vi "Get Instruments.vi"(8 "error in":errorcluster, 10 "Engine":string, 11 "Submodule in":refnum<class "Submodule EOL.lvclass">) -> (0 "error out":errorcluster, 1 "Instrument nodes":refnum<data-value>[](array[refnum]), 2 "Instruments":string[](array[string]), 3 "Submodule out":refnum<class "Submodule EOL.lvclass">)   [LabVIEW 2025, in "Submodule EOL.lvlib" / "Submodule EOL.lvclass"]
uses:
  Submodule EOL.lvclass
  Users/Public/Documents/Sandia National Labs/TSS Plugin/Abstract Engine.lvlibp/Plugin/Abstract/Abstract Instrument/Abstract Instrument.lvclass
  Users/Public/Documents/Sandia National Labs/TSS Plugin/Abstract Engine.lvlibp/Plugin/Abstract/Abstract Engine/Abstract Engine.lvclass
  Users/Public/Documents/Sandia National Labs/TSS Plugin/Abstract Engine.lvlibp/Plugin/Abstract/Engine configuration/Engine configuration.lvclass
  Users/Public/Documents/Sandia National Labs/TSS Plugin/Abstract Engine.lvlibp/Plugin/Abstract/Instrument configuration/Instrument configuration.lvclass
  Users/Public/Documents/Sandia National Labs/TSS Plugin/CEF.lvlibp/Node/ReadParent.vi
  Users/Public/Documents/Sandia National Labs/TSS Plugin/CEF.lvlibp/Node/ReadChildren.vi
  Users/Public/Documents/Sandia National Labs/TSS Plugin/CEF.lvlibp/Node/ReadNodeClass.vi
  Users/Public/Documents/Sandia National Labs/TSS Plugin/Abstract Engine.lvlibp/Plugin/Abstract/Engine configuration/Read Engine Setting.vi
  Users/Public/Documents/Sandia National Labs/TSS Plugin/Abstract Engine.lvlibp/Plugin/Abstract/Instrument configuration/Read Instrument Setting.vi
  Users/Public/Documents/Sandia National Labs/TSS Plugin/CEF.lvlibp/Node/CEF_Node.lvclass
  Users/Public/Documents/Sandia National Labs/TSS Plugin/CEF.lvlibp/serializable configuration/CEF_serializable configuration.lvclass
  Submodule EOL.lvclass/Submodule EOL.ctl
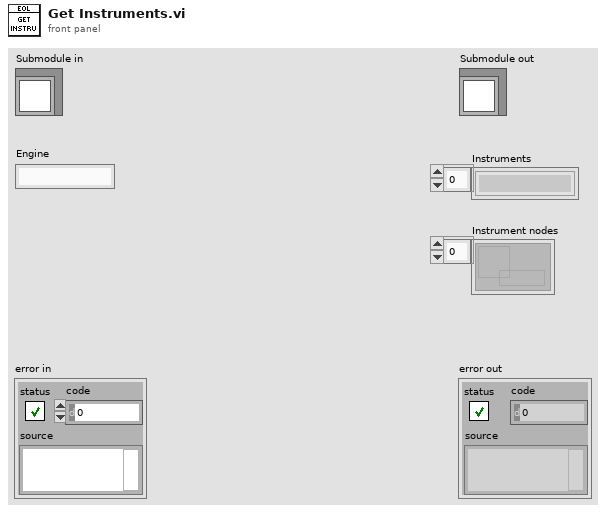
[diagram p1: front panel]
types:
  T1 = typedef "Abstract Engine.lvlibp/Engine configuration.lvclass/Engine Setting.ctl" = cluster{"Enabled":bool, "IP Address":string, "Port":i32, "Description":string, "Type":string, "Version":string}
  T2 = typedef "Abstract Engine.lvlibp/Instrument configuration.lvclass/Default Instrument.ctl" = cluster{"Type":string, "Address":string, "SW Alias":string, "Description":string, "Enabled":bool}
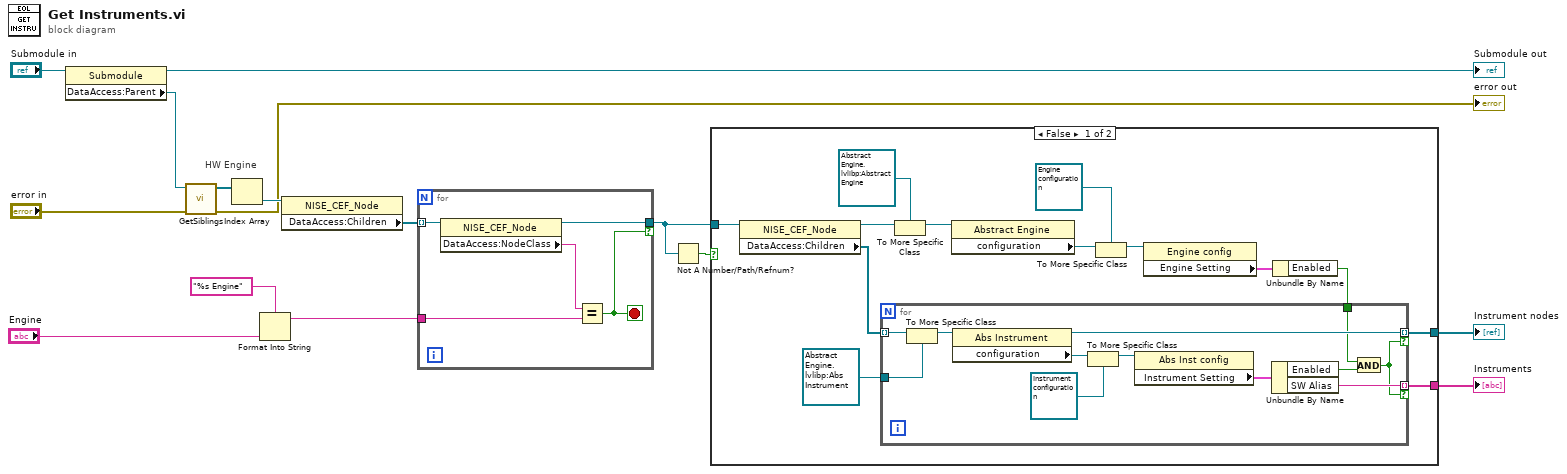
[diagram p0: block diagram]
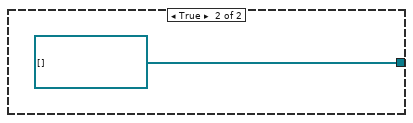
[diagram p2: hidden frame]
diagram:
  # "HW Engine"
  n1 = property class="Submodule"(reference="Submodule in") -> (reference out=→"Submodule out":refnum<class "Submodule EOL.lvclass">, "DataAccess:Parent"=w13:refnum<data-value>)  [unwired: 1 in, 1 out]
  n2 = call "GetSiblings.vi"("error in"="error in", "node in"=w13) -> ("error out"=→"error out":errorcluster, "siblings"=w12:refnum<data-value>[])  [unwired: 8 in]
  n3 = Index Array(array=w12) -> (element=w11:refnum<data-value>)  [unwired: 1 in]
  n4 = Format Into String(format string="%s Engine", "Engine") -> (resulting string=w1:string)  [unwired: 2 in, 1 out]
  n5 = property class="NISE_CEF_Node"(reference=w11) -> ("DataAccess:Children"=w10:refnum<data-value>[])  [unwired: 1 in, 2 out]
  n6 = for {
    tunnel: w10 -> [w20] mode=indexing
    tunnel: [w18] -> w8 if=w17
    tunnel: w1 -> [w16]
    stop <- w17 stop-if-true
    n7 = property class="NISE_CEF_Node"(reference=w20) -> (reference out=w18:refnum<data-value>, "DataAccess:NodeClass"=w19:string)  [unwired: 1 in, 1 out]
    n8 = Equal?(x=w19, y=w16) -> (x = y?=w17:bool)
  }
  n9 = Not A Number/Path/Refnum?(number/path/refnum=w8) -> (NaN/Path/Refnum?=w9:bool)
  n10 = case shown="False" w9 {
    tunnel: w8 -> [w33 _]
    tunnel: [w22 refnum<data-value>[] []] -> w6
    tunnel: [w21 _] -> w4
    frame False {
      n11 = property class="NISE_CEF_Node"(reference=w33) -> (reference out=w32:refnum<data-value>, "DataAccess:Children"=w30:refnum<data-value>[])  [unwired: 1 in, 1 out]
      n12 = To More Specific Class(target class=refnum<data-value> refnum, reference=w32) -> (specific class reference=w24:refnum<data-value>)  [unwired: 1 in, 1 out]
      n13 = property class="Abstract Engine"(reference=w24) -> ("configuration"=w28:refnum<class "CEF_serializable configuration.lvclass">)  [unwired: 1 in, 2 out]
      n14 = To More Specific Class(target class=refnum<class "Engine configuration.lvclass"> refnum ("Abstract Engine.lvlibp:Engine config"), reference=w28) -> (specific class reference=w27:refnum<class "Engine configuration.lvclass">)  [unwired: 1 in, 1 out]
      n15 = property class="Engine config"(reference=w27) -> ("Engine Setting"=w26:T1)  [unwired: 1 in, 2 out]
      n16 = Unbundle By Name(w26) -> ("Enabled"=w23:bool)
      n17 = for {
        tunnel: w30 -> [w45] mode=indexing
        tunnel: refnum<data-value> refnum ("target class") -> [w44]
        tunnel: [w38] -> w21 mode=indexing if=w34
        tunnel: [w37] -> w22 mode=indexing if=w34
        tunnel: w23 -> [w36]
        n18 = To More Specific Class(target class=w44, reference=w45) -> (specific class reference=w43:refnum<data-value>)  [unwired: 1 in, 1 out]
        n19 = property class="Abs Instrument"(reference=w43) -> (reference out=w37:refnum<data-value>, "configuration"=w42:refnum<class "CEF_serializable configuration.lvclass">)  [unwired: 1 in, 1 out]
        n20 = To More Specific Class(target class=refnum<class "Instrument configuration.lvclass"> refnum ("Abstract Engine.lvlibp:Abs Inst config"), reference=w42) -> (specific class reference=w40:refnum<class "Instrument configuration.lvclass">)  [unwired: 1 in, 1 out]
        n21 = property class="Abs Inst config"(reference=w40) -> ("Instrument Setting"=w39:T2)  [unwired: 1 in, 2 out]
        n22 = Unbundle By Name(w39) -> ("Enabled"=w35:bool, "SW Alias"=w38:string)
        n23 = And(x=w36, y=w35) -> (x .and. y?=w34:bool)
      }
    }
    frame True {
    }
  }
  "Instruments" <- w4
  "Instrument nodes" <- w6
